vi "ProducerConsumer.vi"() -> ()   [LabVIEW 2022 SP3]
doc: "Use this template to build a producer/consumer design pattern. Use this template when you need to execute a process, such as data analysis, when a data source, such as a triggered acquisition, produces data at an uneven rate and you need to execute the process when the data becomes available."
uses:
  <vilib>/DAQmx/read.llb/DAQmx Read (Analog 1D Wfm NChan NSamp).vi
  <vilib>/DAQmx/miscellaneous.llb/DAQmx Fill In Error Info.vi
  <resource>/objmgr/daqmx.rc
panel:
  out "Waveform Graph":waveform(dbl)[](graph)
  in  "stop":bool
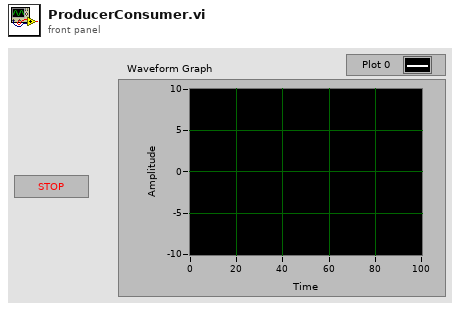
[diagram p1: front panel]
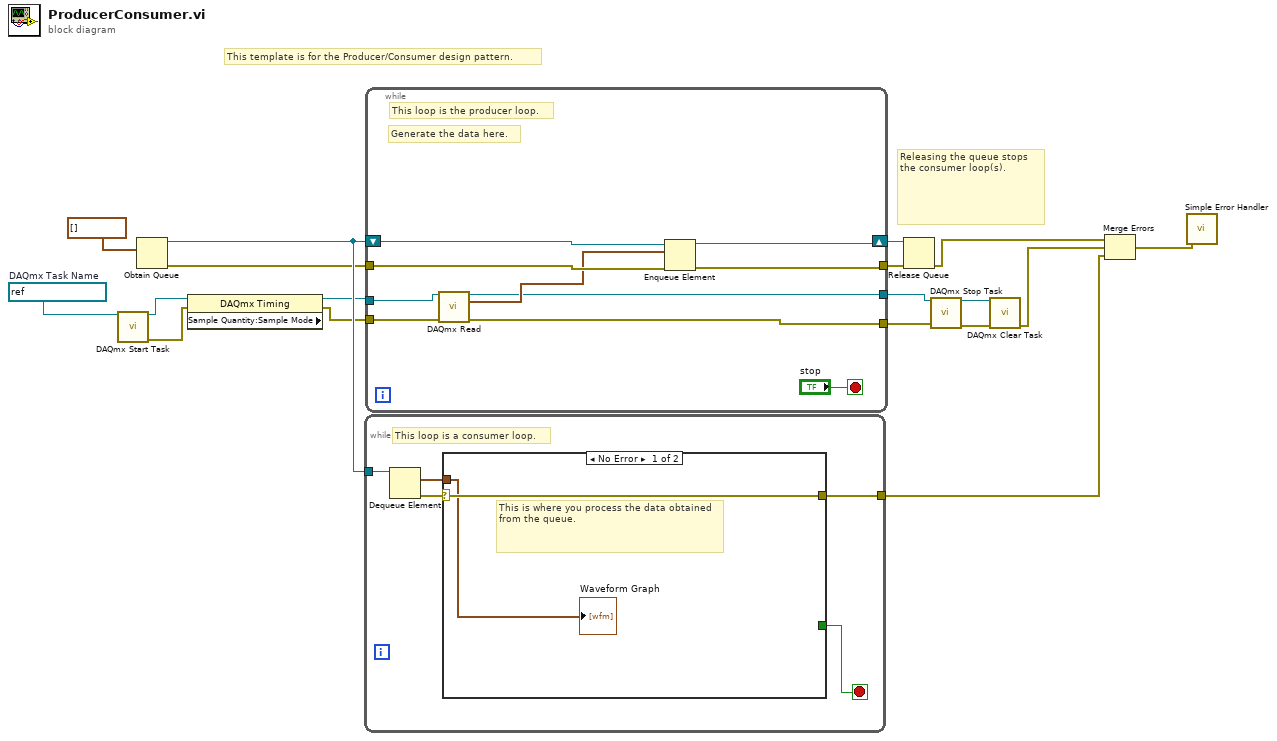
[diagram p0: block diagram]
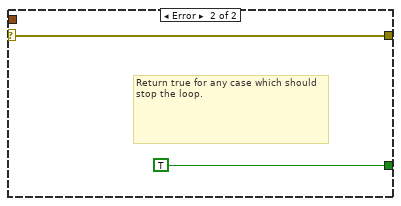
[diagram p2: hidden frame]
diagram:
  w14 = refnum<k21> "FTS2_120VAC"  # DAQmx Task Name
  # "Releasing the queue stops the consumer loop(s)."
  # "This template is for the Producer/Consumer design pattern."
  n1 = call <vilib>:"DAQmx Start Task.vi"("task/channels in"=w14) -> ("task out"=w15:refnum<k21>, "error out"=w4:errorcluster)  [unwired: 13 in]
  n2 = Obtain Queue(element data type=waveform(dbl)[] [] ("Array")) -> (queue out=w18:refnum<queue>, error out=w5:errorcluster)  [unwired: 4 in, 1 out]
  n3 = property class="DAQmx Timing" props=["Sample Quantity:Sample Mode"](reference=w15, error in=w4) -> (reference out=w13:refnum<k21>, error out=w3:errorcluster)  [unwired: 1 out]
  n4 = while {
    tunnel: w18 -> [w23]
    tunnel: [w19] -> w2
    stop <- w20 stop-if-true
    # "This loop is a consumer loop."
    n5 = Dequeue Element(queue=w23) -> (element=w21:waveform(dbl)[], error out=w22:errorcluster)  [unwired: 2 in, 2 out]
    n6 = case shown="No Error" w22 {
      selector: w22 -> [w25 w26]
      tunnel: w21 -> [w24 _]
      tunnel: [_ TRUE] -> w20
      tunnel: [w25 w26] -> w19
      frame No Error {
        # "This is where you process the data obtained from the queue."
        "Waveform Graph" <- w24
      }
      frame Error {
        # "Return true for any case which should stop the loop."
      }
    }
  }
  n7 = while {
    shift-right: [w35] -> w17
    shift-left: w18 -> [w36]
    tunnel: w13 -> [w31]
    tunnel: w3 -> [w30]
    tunnel: [w29] -> w10
    tunnel: w5 -> [w34]
    tunnel: [w33] -> w16
    tunnel: [w28] -> w1
    stop <- "stop" stop-if-true
    # "Generate the data here."
    # "This loop is the producer loop."
    n8 = call-poly <vilib>:"DAQmx Read.vi"("task/channels in"=w31, "error in"=w30) -> ("task out"=w28:refnum<k21>, "data"=w32:waveform(dbl)[], "error out"=w29:errorcluster)  [unwired: 11 in]
    n9 = Enqueue Element(queue=w36, element=w32, error in (no error)=w34) -> (queue out=w35:refnum<queue>, error out=w33:errorcluster)  [unwired: 1 in, 1 out]
  }
  n10 = Release Queue(queue=w17, error in (no error)=w16) -> (error out=w9:errorcluster)  [unwired: 1 in, 2 out]
  n11 = call <vilib>:"DAQmx Stop Task.vi"("task/channels in"=w1, "error in"=w10) -> ("task out"=w12:refnum<k21>, "error out"=w11:errorcluster)  [unwired: 12 in]
  n12 = call <vilib>:"DAQmx Clear Task.vi"("task in"=w12, "error in"=w11) -> ("error out"=w8:errorcluster)  [unwired: 13 in]
  n13 = Merge Errors(w9, w8, w2) -> (w7:errorcluster)
  n14 = call <vilib>:"Simple Error Handler.vi"("error in (no error)"=w7) -> ()  [unwired: 4 in, 5 out]
